vi "Measure vs B2Dv14.vi"() -> ()   [LabVIEW 2009]
doc: "This VI is an example operator panel.\n\nThe VI contains a table for the field values that may be configured manually, or loaded by checking the \"Prompt for File\" box. The data file should contain 3 columns of data, with each column delimited by a tab character.\n\nBefore the VI is executed, set the desired field units and coordinate system. Once the VI is started, follow the directions in the STATUS indicator to operate. Once a field value is achieved, it will be held indefinitely with no user intervention.\n\nThe present field is displayed in the selected units and coordinate system. The present field is queried once per second.\n\nIf a field point is specified that is outside the limits for the magnet, the VI will abort execution."
uses:
  <vilib>/Utility/file.llb/Read From Spreadsheet File (DBL).vi
panel:
  in  "Choose AH (2550 - 2700)":bool=TRUE
  in  "PID off":bool
  in  "Go to zero and SH off":bool=TRUE
  in  "Port Num- TRBridge":string="7"
  in  "GPIB SIM900":string="2"
  in  "TempSensor":bool
  in  "AH":bool=TRUE
  in  "GPIB HP 2":string="13"
  in  "Wait between \nVectors":bool
  in  "Change\nPID\n(DetermineSIMPID.vi)":bool
  in  "Wait between \nVectors (ms)":u32=3000
  in  "X Axis":enum16{"B", "phi"}(ring)
  in  "Y Axis":T1(ring)=enum."HP (V)2"
  out "measured data":dbl[][](array[numeric])
  out "XY Graph":T2(graph)
  in  "Notes:":string="test" caption="Notizen:"
  out "Messfile Refnum":refnum<file>
  in  "Measurement File":path=path "D:/UserData/fherzog/FH-4069-5B/test.txt"
  in  "Sample name:":string="FH-4069-5B"
  in  "HP 1":bool
  in  "GPIB HP":string="13"
  in  "HP 2":bool
  in  "LI 3":bool
  in  "GPIB L 3":string="8"
  in  "LI 2":bool
  in  "GPIB L 2":string="8"
  in  "LI 1":bool
  in  "GPIB L 1":string="8"
  out "Number of lines":i32=4
  in  "Operation":u16(ring)=1 items=["Stepwise", "Continous"]
  out "Ramp Rate along Vector (T/min)":dbl=0.060000000000000005 format="%.3f"
  out "Current Ramp Rate Z (T/min)":dbl=0.05908831630883079 format="%.3f"
  out "Current Ramp Rate Y (T/min)":dbl=0.010419734919255939 format="%.3f"
  in  "User defined Ramp Rate (T/min)":bool=TRUE
  in  "User defined Ramp Rate (T/min)":dbl=0.06 format="%.3f"
  in  "Z-Axis Communications Config":T3={"GPIB address"=22, "GPIB bus"=1, "connection ID"=refnum, "IP"="111.111.111.1", "Active Comm Interface"=0, "Serial Port"="", "Programmer Type"=0} {"Programmer Type" items=["Model 430", "Model 420"]; "Active Comm Interface" items=["TCP/IP (Model 430 Only)", "RS232", "IEEE488"]}
  in  "Max Ramp Rate - Y Axis (A/s)":dbl=0.055 format="%.3f"
  in  "Max Ramp Rate - Z Axis (A/s)":dbl=0.19 format="%.3f"
  in  "Magnitude Limit (kG)":dbl=45.1 format="%.3f"
  in  "Y-Axis Communications Config":T3={"GPIB address"=22, "GPIB bus"=1, "connection ID"=refnum, "IP"="111.111.111.2", "Active Comm Interface"=0, "Serial Port"="", "Programmer Type"=0} {"Programmer Type" items=["Model 430", "Model 420"]; "Active Comm Interface" items=["TCP/IP (Model 430 Only)", "RS232", "IEEE488"]}
  out "Cartesian Display (T)":T4={"Y-Axis Field (T)"=-0.08586, "Z-Axis Field (T)"=0.49363} {"Z-Axis Field (T)" format="%.3f"; "Y-Axis Field (T)" format="%.3f"}
  in  "Starting index":i32=4
  in  "Normal color":u32(colorbox)=11711154
  in  "Highlight color":u32(colorbox)=16711680
  in  "Prompt for File?":bool
  out "Continue Execution?":bool=TRUE
  out "error out":T5
  in  "error in":T5
  out "STATUS":string="Holding at current vector. Set Ramping Mode to NEXT VECTOR to continue."
  in  "Ramping Control":u16(ring)=2 items=["NEXT VECTOR", "RAMPING", "HOLDING", "PAUSE", "ZERO"]
  out "Cartesian Display (kG)":T6 {"Z-Axis Field (kG)" format="%.3f"; "Y-Axis Field (kG)" format="%.3f"}
  in  "Field Values":string[][](table)=[["3.5", "100"], ["8.1", "100"], ["3.5", "100"], ["8.1", "100"]]
  out "Switch Heaters":bool=TRUE
  out "Polar Display (T)":T7 {"Field Magnitude (T)" format="%.3f"; "q (degrees)" format="%.3f"}
  out "Polar Display (kG)":T8 {"Field Magnitude (kG)" format="%.3f"; "q (degrees)" format="%.3f"}
  in  "Coordinate System":u16(ring)=1 items=["Cartesian", "Polar"]
  in  "Magnetic Field Units":u16(ring)=1 items=["kG", "Tesla"]
  # "kontinuirliche Messung mit PID off bei 0, geht nur im Cartesian mode!"
  # "Measurement Display"
  # "Measurement Settings"
  # "Magnet Settings"
  # "Max Ramp Rate z: 1.27 T/min\nMax Ramp Rate y: 0.17 T/min"
  # "Devices"
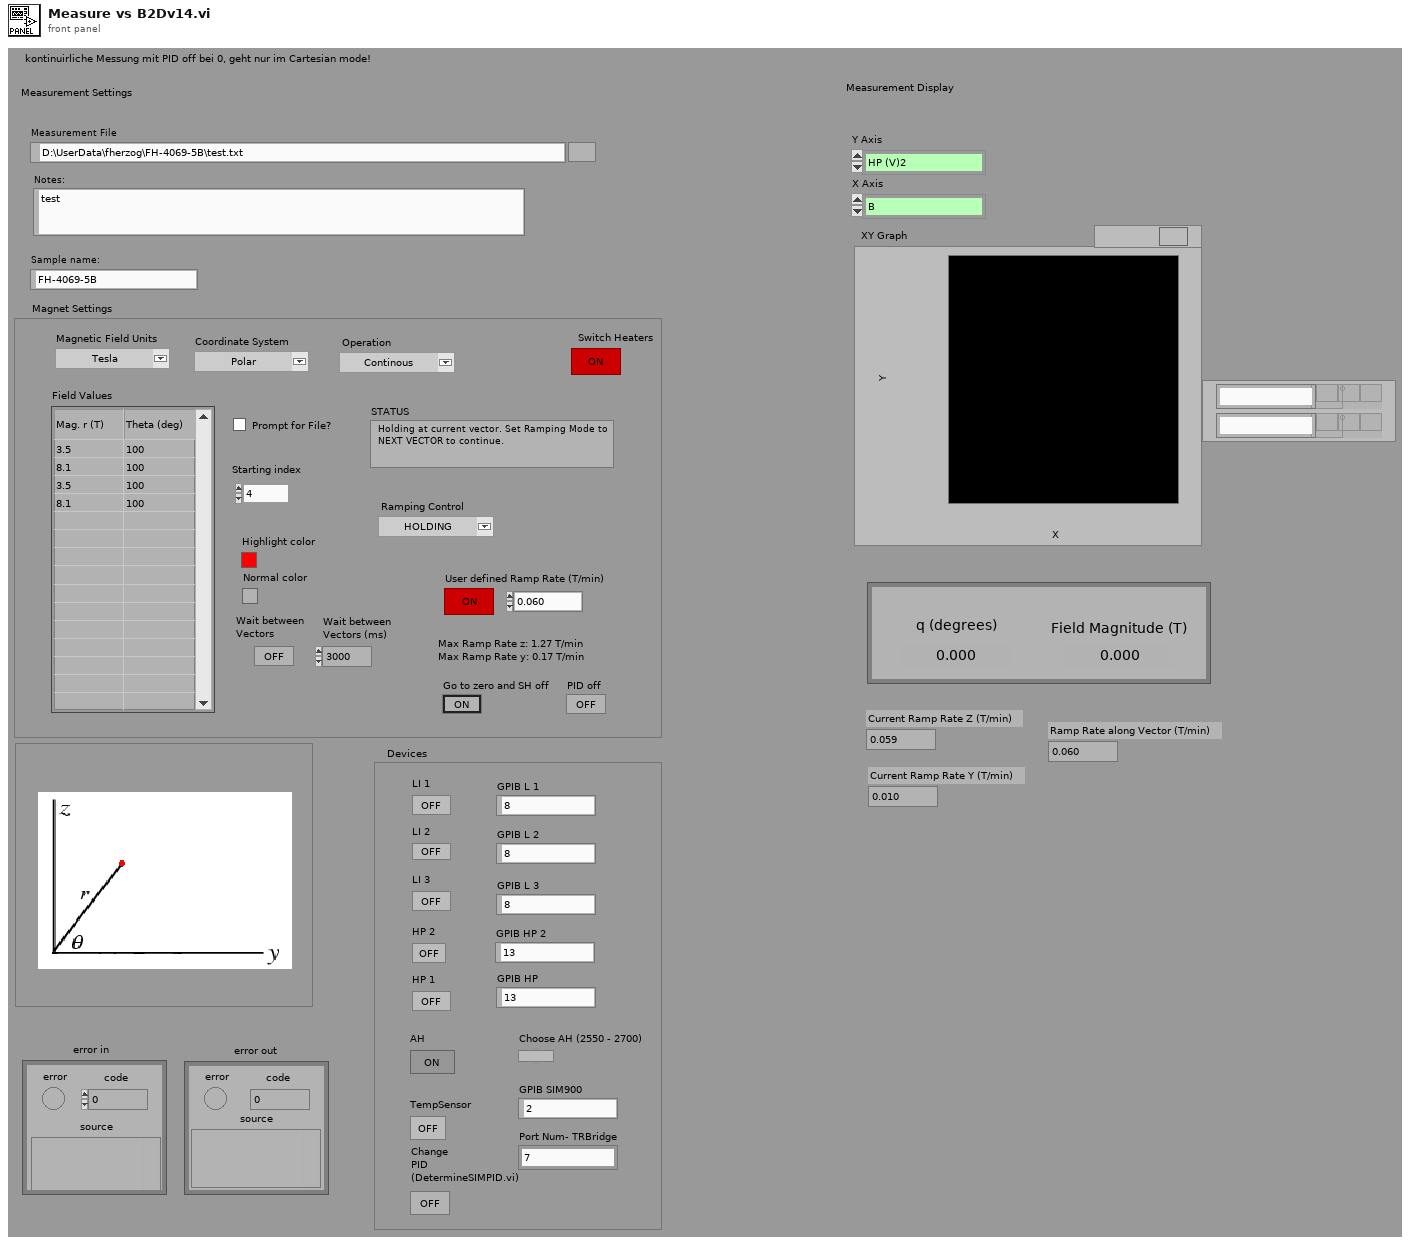
[diagram p1: front panel]
types:
  T1 = enum16{"B", "phi", "LI 1 Vx", "LI 1 Vy", "LI 2 Vx", "LI 2 Vy", "LI 3 Vx", "LI 3 Vy", "LI 4 Vx", "LI 4 Vy", "HP (V)", "HP (V)2", "AH C (pF)", "AH loss", "T (Ohms)", "Timestamp"}
  T2 = cluster{"measured data":dbl[], "measured data":dbl[]}
  T3 = cluster{"GPIB address":i16, "GPIB bus":i16, "connection ID":refnum<k5>, "IP":string, "Active Comm Interface":u16, "Serial Port":refnum<visa-resource-name>, "Programmer Type":u16}
  T4 = cluster{"Y-Axis Field (T)":dbl, "Z-Axis Field (T)":dbl}
  T5 = cluster{"error":bool, "code":i32, "source":string}
  T6 = cluster{"Y-Axis Field (kG)":dbl, "Z-Axis Field (kG)":dbl}
  T7 = cluster{"q (degrees)":dbl, "Field Magnitude (T)":dbl}
  T8 = cluster{"q (degrees)":dbl, "Field Magnitude (kG)":dbl}
  T9 = enum16{"", "RAMPING", "HOLDING", "PAUSED", "MANUAL UP", "MANUAL DOWN", "ZEROING CURRENT", "QUENCH DETECTED", "HEATING SWITCH"}
  T10 = enum16{"", "RAMPING", "HOLDING", "PAUSED", "MANUAL UP", "MANUAL DOWN", "ZEROING CURRENT", "QUENCH DETECTED", "HEATING SWITCH", "AT ZER0", "COOLING SWITCH"}
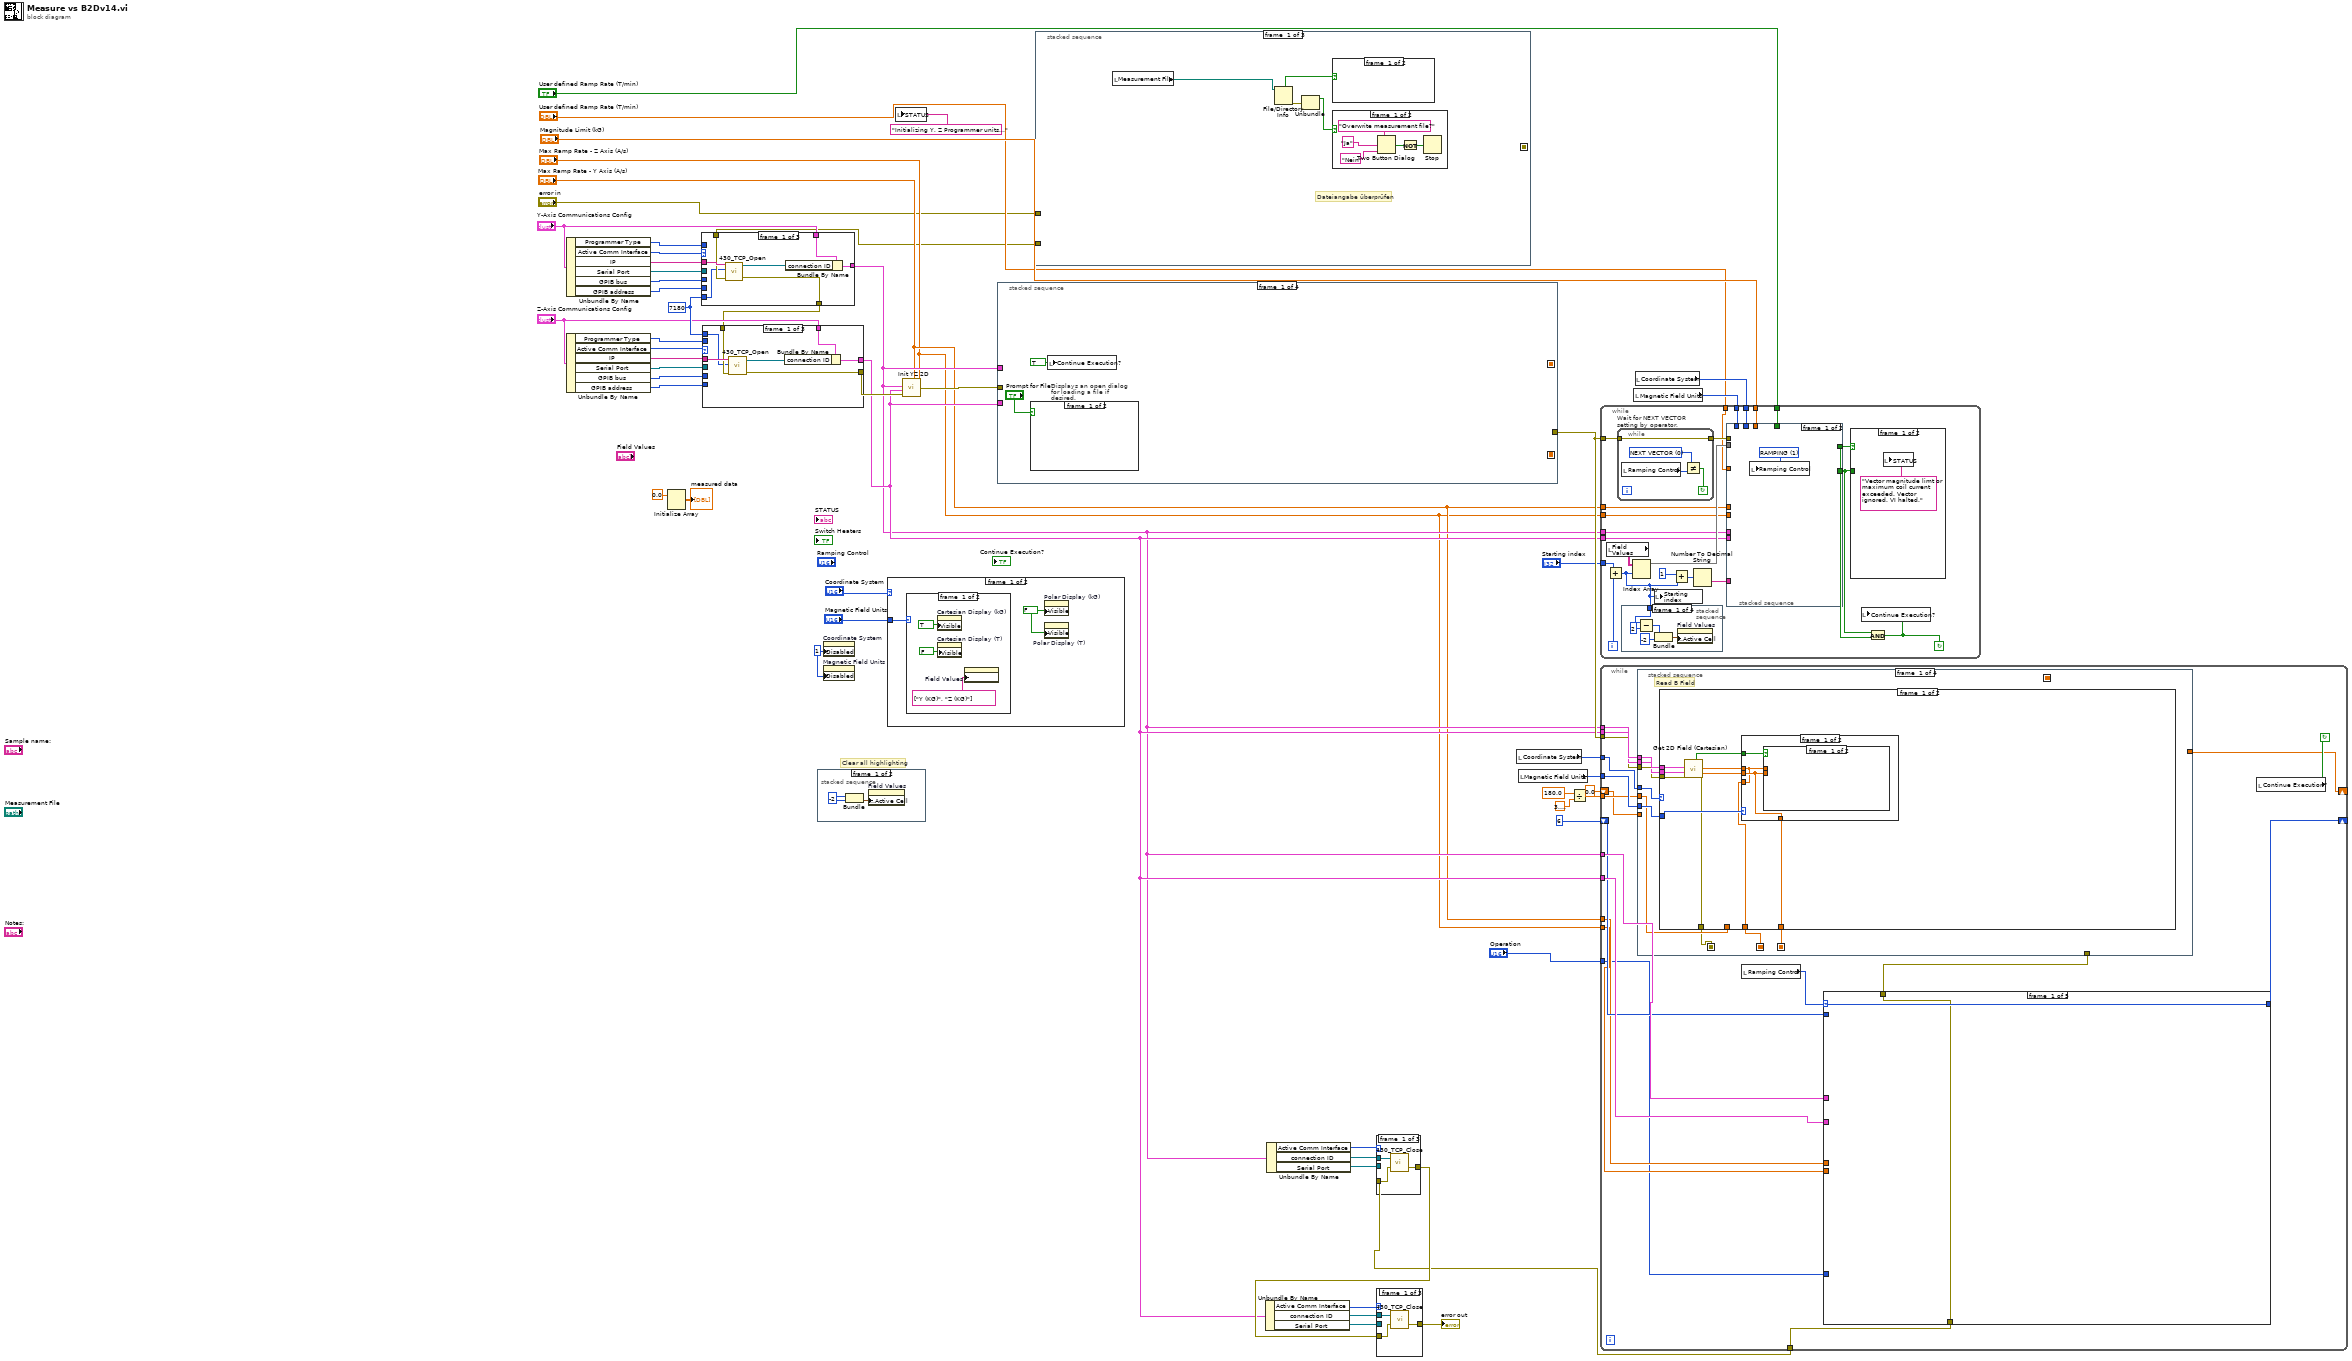
[diagram p0: block diagram]
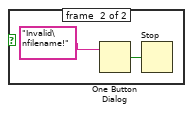
[diagram p3: hidden frame]
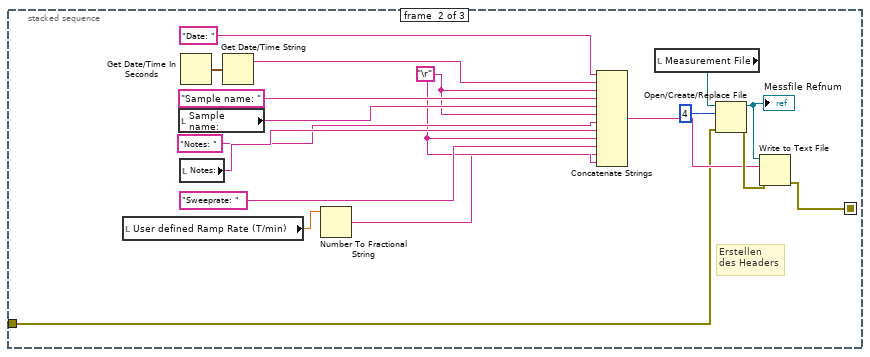
[diagram p4: hidden frame]
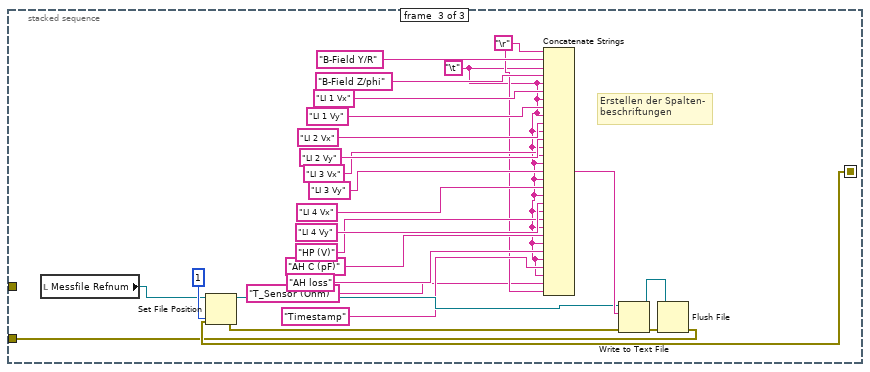
[diagram p5: hidden frame]
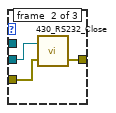
[diagram p6: hidden frame]
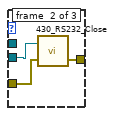
[diagram p8: hidden frame]
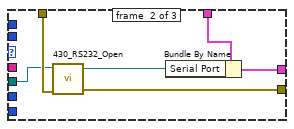
[diagram p10: hidden frame]
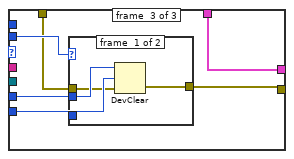
[diagram p11: hidden frame]
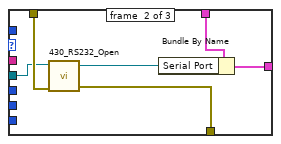
[diagram p13: hidden frame]
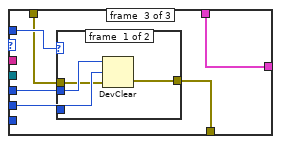
[diagram p14: hidden frame]
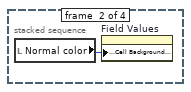
[diagram p16: hidden frame]
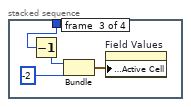
[diagram p17: hidden frame]
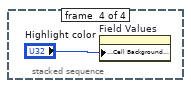
[diagram p18: hidden frame]
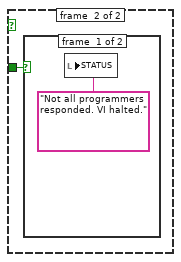
[diagram p19: hidden frame]
diagram:
  w39 = 7180 ("TCP Port")
  w52 = u8 1 ("Write Attribute")
  # "Clear all highlighting"
  n1 = Unbundle By Name("Z-Axis Communications Config") -> ("Programmer Type"=w15:u16, "Active Comm Interface"=w38:u16, "IP"=w35:string, "Serial Port"=w34:refnum<visa-resource-name>, "GPIB bus"=w14:i16, "GPIB address"=w13:i16)
  n2 = Unbundle By Name("Y-Axis Communications Config") -> ("Programmer Type"=w9:u16, "Active Comm Interface"=w37:u16, "IP"=w36:string, "Serial Port"=w33:refnum<visa-resource-name>, "GPIB bus"=w10:i16, "GPIB address"=w11:i16)
  n3 = Initialize Array(0.0 ("element")) -> (→"measured data":dbl[][])  [unwired: 2 in]
  n4 = stacked-sequence {
    frame #0 {
      w55 = -2
      n5 = Bundle(w55, w55) -> (w56:cluster{i32, i32})  [unwired: 1 in]
      n6 = property on="Field Values" class="Tbl (strict)"("Active Cell:Active Cell"=w56) -> ()  [unwired: 2 in, 2 out]
    }
    frame #1 {
      n7 = property on="Field Values" class="Tbl (strict)"("Active Cell:Cell Background Color"="Normal color") -> ()  [unwired: 2 in, 2 out]
    }
  }
  n8 = property on="Coordinate System" class="Ring (strict)"("Disabled"=w52) -> ()  [unwired: 2 in, 2 out]
  n9 = property on="Magnetic Field Units" class="Ring (strict)"("Disabled"=w52) -> ()  [unwired: 2 in, 2 out]
  n10 = case shown="1" "Coordinate System" {
    tunnel: "Magnetic Field Units" -> [w59 w67]
    frame #0 {
      w58 = FALSE ("Write Attribute")
      (unwired) FALSE ("Write Attribute")
      (unwired) TRUE ("Write Attribute")
      n11 = case shown="1" w59 {
        frame #0 {
          n12 = property on="Cartesian Display (kG)" class="Cluster (strict)"("Visible"=TRUE ("Write Attribute")) -> ()  [unwired: 2 in, 2 out]
          n13 = property on="Cartesian Display (T)" class="Cluster (strict)"("Visible"=FALSE ("Write Attribute")) -> ()  [unwired: 2 in, 2 out]
          n14 = property on="Field Values" class="Tbl (strict)"("Column Header Strings[]"=string[] ["Y (KG)", "Z (KG)"] ("Write Attribute")) -> ()  [unwired: 2 in, 2 out]
        }
        frame #1 {
          n15 = property on="Cartesian Display (kG)" class="Cluster (strict)"("Visible"=FALSE ("Write Attribute")) -> ()  [unwired: 2 in, 2 out]
          n16 = property on="Cartesian Display (T)" class="Cluster (strict)"("Visible"=TRUE ("Write Attribute")) -> ()  [unwired: 2 in, 2 out]
          n17 = property on="Field Values" class="Tbl (strict)"("Column Header Strings[]"=string[] ["Y (T)", "Z (T)"] ("Write Attribute")) -> ()  [unwired: 2 in, 2 out]
        }
      }
      n18 = property on="Polar Display (kG)" class="Clust (strict)"("Visible"=w58) -> ()  [unwired: 2 in, 2 out]
      n19 = property on="Polar Display (T)" class="Clust (strict)"("Visible"=w58) -> ()  [unwired: 2 in, 2 out]
    }
    frame #1 {
      (unwired) FALSE ("Write Attribute")
      (unwired) TRUE ("Write Attribute")
      w66 = FALSE ("Write Attribute")
      n20 = case shown="1" w67 {
        frame #0 {
          n21 = property on="Polar Display (kG)" class="Clust (strict)"("Visible"=TRUE ("Write Attribute")) -> ()  [unwired: 2 in, 2 out]
          n22 = property on="Polar Display (T)" class="Clust (strict)"("Visible"=FALSE ("Write Attribute")) -> ()  [unwired: 2 in, 2 out]
          n23 = property on="Field Values" class="Tbl (strict)"("Column Header Strings[]"=string[] ["Mag. r (KG)", "Theta (deg)"] ("Write Attribute")) -> ()  [unwired: 2 in, 2 out]
        }
        frame #1 {
          n24 = property on="Polar Display (kG)" class="Clust (strict)"("Visible"=FALSE ("Write Attribute")) -> ()  [unwired: 2 in, 2 out]
          n25 = property on="Polar Display (T)" class="Clust (strict)"("Visible"=TRUE ("Write Attribute")) -> ()  [unwired: 2 in, 2 out]
          n26 = property on="Field Values" class="Tbl (strict)"("Column Header Strings[]"=string[] ["Mag. r (T)", "Theta (deg)"] ("Write Attribute")) -> ()  [unwired: 2 in, 2 out]
        }
      }
      n27 = property on="Cartesian Display (kG)" class="Cluster (strict)"("Visible"=w66) -> ()  [unwired: 2 in, 2 out]
      n28 = property on="Cartesian Display (T)" class="Cluster (strict)"("Visible"=w66) -> ()  [unwired: 2 in, 2 out]
    }
  }
  n29 = local write "STATUS"("Initializing Y, Z Programmer units..." ("STATUS")) -> ()
  n30 = stacked-sequence {
    seq-local: [_ w85 _] -> [_ _ w110]
    tunnel: "error in" -> [_ w86 _]
    tunnel: [_ _ w109] -> w4
    frame #0 {
      # "Dateiangabe überprüfen"
      n31 = local read "Measurement File"() -> (w77:path)
      n32 = File/Directory Info(path=w77) -> (directory=w75:bool, error out=w76:errorcluster)  [unwired: 1 in, 5 out]
      n33 = Unbundle(w76) -> ("status"=w74:bool)  [unwired: 2 out]
      n34 = case shown="False" w75 {
        frame #0 {
        }
        frame #1 {
          n35 = One Button Dialog(message="Invalid\nfilename!") -> (true=w83:bool)  [unwired: 1 in]
          n36 = Stop(stop? (T)=w83) -> ()
        }
      }
      n37 = case shown="False" w74 {
        frame #0 {
          n38 = Two Button Dialog(message="Overwrite measurement file?", 1:"Nein", 2:"Ja") -> (T button?=w79:bool)
          n39 = Not(x=w79) -> (.not. x?=w78:bool)
          n40 = Stop(stop? (T)=w78) -> ()
        }
        frame #1 {
        }
      }
    }
    frame #1 {
      w89 = "\r"
      # "Erstellen\ndes Headers"
      n41 = local read "User defined Ramp Rate (T/min)"() -> (w88:dbl)
      n42 = local read "Sample name:"() -> (w95:string)
      n43 = local read "Notes:"() -> (w97:string)
      n44 = Get Date/Time In Seconds() -> (seconds since 1Jan1904=w91:timestamp)
      n45 = Get Date/Time String(seconds (now)=w91) -> (date string=w93:string)  [unwired: 2 in, 1 out]
      n46 = Number To Fractional String(number=w88) -> (F-format string=w87:string)  [unwired: 3 in]
      n47 = Concatenate Strings("Date: ", w93, w89, "Sample name: ", w95, w89, "Notes: ", w97, w89, "Sweeprate: ", w87, w89) -> (w101:string)
      n48 = local read "Measurement File"() -> (w98:path)
      n49 = Open/Create/Replace File(file path (use dialog)=w98, error in=w86, operation (0:open)=4) -> (refnum out=w100:refnum<file>, error out=w102:errorcluster)  [unwired: 3 in, 1 out]
      "Messfile Refnum" <- w100
      n50 = Write to Text File(file (use dialog)=w100, text=w101, error in=w102) -> (error out=w85:errorcluster)  [unwired: 1 in, 2 out]
    }
    frame #2 {
      w104 = "\t"
      w105 = "\r"
      # "Erstellen der Spalten-\nbeschriftungen"
      n51 = local read "Messfile Refnum"() -> (w117:refnum<file>)
      n52 = Set File Position(refnum=w117, from (0:start)=1, error in=w110) -> (refnum out=w123:refnum<file>, error out=w125:errorcluster)  [unwired: 1 in]
      n53 = Concatenate Strings(w105, "B-Field Y/R", w104, "B-Field Z/phi", w104, "LI 1 Vx", w104, "LI 1 Vy", w104, "LI 2 Vx", w104, "LI 2 Vy", w104, "LI 3 Vx", w104, "LI 3 Vy", w104, "LI 4 Vx", w104, "LI 4 Vy", w104, "HP (V)", w104, "AH C (pF)" ("string"), w104, "AH loss" ("string"), w104, "Timestamp", w104, "T_Sensor (Ohm)" ("string"), w105) -> (w124:string)
      n54 = Write to Text File(file (use dialog)=w123, text=w124, error in=w125) -> (refnum out=w127:refnum<file>, error out=w126:errorcluster)  [unwired: 1 in, 1 out]
      n55 = Flush File(refnum=w127, error in=w126) -> (error out=w109:errorcluster)  [unwired: 1 out]
    }
  }
  n56 = case shown="0, Default" w37 {
    tunnel: w36 -> [w135 _ _]
    tunnel: w4 -> [w134 w141 w143]
    tunnel: "Y-Axis Communications Config" -> [w133 w136 w147]
    tunnel: [w131 w139 w147] -> w22
    tunnel: [w130 w140 w142] -> w12
    tunnel: w39 -> [w129 _ _]
    tunnel: w33 -> [_ w137 _]
    tunnel: w11 -> [_ _ w146]
    tunnel: w10 -> [_ _ w145]
    tunnel: w9 -> [_ _ w144]
    frame #0 {
      n57 = call <userlib>:"430_TCP_Open.vi"("IP Address"=w135, "TCP Port"=w129, "error in (no error)"=w134) -> ("connection ID"=w132:refnum<k5>, "error out"=w130:errorcluster)  [unwired: 3 in, 1 out]
      n58 = Bundle By Name(cluster=w133, "connection ID"=w132) -> (w131:T3)
    }
    frame #1 {
      n59 = call <userlib>:"430_RS232_Open.vi"("VISA resource name"=w137, "error in (no error)"=w141) -> ("VISA resource name out"=w138:refnum<visa-resource-name>, "error out"=w140:errorcluster)  [unwired: 5 in]
      n60 = Bundle By Name(cluster=w136, "Serial Port"=w138) -> (w139:T3)
    }
    frame #2 {
      n61 = case shown="1" w144 {
        tunnel: w145 -> [w151 _]
        tunnel: w146 -> [w150 _]
        tunnel: w143 -> [w149 w152]
        tunnel: [w148 w152] -> w142
        frame #0 {
          n62 = DevClear(2:w149, 3:w150, 4:w151) -> (0:w148:errorcluster)  [unwired: 1 out]
        }
        frame #1 {
        }
      }
    }
  }
  n63 = case shown="0, Default" w38 {
    tunnel: w35 -> [w159 _ _]
    tunnel: w12 -> [w158 w165 w167]
    tunnel: [w157 w164 w166] -> w32
    tunnel: "Z-Axis Communications Config" -> [w156 w162 w171]
    tunnel: [w154 w163 w171] -> w23
    tunnel: w39 -> [w153 _ _]
    tunnel: w34 -> [_ w160 _]
    tunnel: w15 -> [_ _ w170]
    tunnel: w14 -> [_ _ w169]
    tunnel: w13 -> [_ _ w168]
    frame #0 {
      n64 = call <userlib>:"430_TCP_Open.vi"("IP Address"=w159, "TCP Port"=w153, "error in (no error)"=w158) -> ("connection ID"=w155:refnum<k5>, "error out"=w157:errorcluster)  [unwired: 3 in, 1 out]
      n65 = Bundle By Name(cluster=w156, "connection ID"=w155) -> (w154:T3)
    }
    frame #1 {
      n66 = call <userlib>:"430_RS232_Open.vi"("VISA resource name"=w160, "error in (no error)"=w165) -> ("VISA resource name out"=w161:refnum<visa-resource-name>, "error out"=w164:errorcluster)  [unwired: 5 in]
      n67 = Bundle By Name(cluster=w162, "Serial Port"=w161) -> (w163:T3)
    }
    frame #2 {
      n68 = case shown="0, Default" w170 {
        tunnel: w169 -> [w175 _]
        tunnel: w168 -> [w174 _]
        tunnel: w167 -> [w173 w176]
        tunnel: [w172 w176] -> w166
        frame #0 {
          n69 = DevClear(2:w173, 3:w174, 4:w175) -> (0:w172:errorcluster)  [unwired: 1 out]
        }
        frame #1 {
        }
      }
    }
  }
  n70 = call <userlib>:"Init YZ 2D.vi"("Max Ramp Rate Z-axis"="Max Ramp Rate - Z Axis (A/s)", "Max Ramp Rate Y-axis"="Max Ramp Rate - Y Axis (A/s)", "error in"=w32, "Z-Axis Communications Config"=w23, "Y-Axis Communications Config"=w22) -> ("error out"=w50:T5)  [unwired: 5 in]
  n71 = stacked-sequence {
    seq-local: [_ w184 _ _] -> [_ _ w231 _]
    seq-local: [_ w183 _ _] -> [_ _ w230 _]
    tunnel: w23 -> [_ w186 _ _]
    tunnel: w50 -> [_ w187 _ _]
    tunnel: [_ w182 _ _] -> w46
    tunnel: w22 -> [_ w185 _ _]
    frame #0 {
      n72 = case "Displays an open dialog for loading a file if desired." shown="True" "Prompt for File?" {
        frame #0 {
        }
        frame #1 {
          n73 = call-poly <vilib>:"Read From Spreadsheet File.vi"() -> ("all rows"=w181:dbl[][])  [unwired: 7 in, 4 out]
          n74 = Number To Fractional String(number=w181, precision (6)=i16 4) -> (F-format string=w180:string[][])  [unwired: 2 in]
          n75 = local write "Field Values"(w180) -> ()
        }
      }
      n76 = local write "Continue Execution?"(TRUE ("Continue Execution?")) -> ()
    }
    frame #1 {
      w195 = u16 3 items=["NEXT VECTOR", "RAMPING", "HOLDING", "PAUSE", "ZERO"] ("Ramping Control")
      n77 = call <userlib>:"Get Switch Present.vi"("error in"=w187, "Communications Config"=w185) -> ("error out"=w191:T5, "Switch Present?"=w192:bool)
      n78 = case shown="True" w192 {
        tunnel: w191 -> [w213 w222]
        tunnel: w185 -> [_ w215]
        tunnel: [0.0 w219] -> w183
        tunnel: [w213 w221] -> w190
        frame #0 {
        }
        frame #1 {
          n79 = call <userlib>:"Get Switch Heater Time.vi"("error in"=w222, "Communications Config"=w215) -> ("error out"=w218:T5, "Switch Heating Time (secs)"=w220:dbl)
          n80 = call <userlib>:"Get Switch Heater.vi"("error in"=w218, "Communications Config"=w215) -> ("error out"=w217:T5, "Switch Heater Indicator"=w216:bool)
          n81 = case shown="False" w216 {
            tunnel: [w227 w228] -> w221
            tunnel: w220 -> [w225 _]
            tunnel: [w225 0.0] -> w219
            tunnel: w217 -> [w223 w228]
            tunnel: w215 -> [w224 _]
            frame #0 {
              n82 = call <userlib>:"Set Switch Heater.vi"("error in"=w223, "Switch Heater Control"=TRUE, "Communications Config"=w224) -> ("error out"=w227:T5)
            }
            frame #1 {
            }
          }
        }
      }
      n83 = call <userlib>:"Get Switch Present.vi"("error in"=w190, "Communications Config"=w186) -> ("error out"=w188:T5, "Switch Present?"=w189:bool)
      n84 = case shown="True" w189 {
        tunnel: w188 -> [w196 w205]
        tunnel: w186 -> [_ w198]
        tunnel: [0.0 w202] -> w184
        tunnel: [w196 w204] -> w182
        frame #0 {
        }
        frame #1 {
          n85 = call <userlib>:"Get Switch Heater Time.vi"("error in"=w205, "Communications Config"=w198) -> ("error out"=w201:T5, "Switch Heating Time (secs)"=w203:dbl)
          n86 = call <userlib>:"Get Switch Heater.vi"("error in"=w201, "Communications Config"=w198) -> ("error out"=w200:T5, "Switch Heater Indicator"=w199:bool)
          n87 = case shown="False" w199 {
            tunnel: [w206 w211] -> w204
            tunnel: w203 -> [w209 _]
            tunnel: [w209 0.0] -> w202
            tunnel: w200 -> [w207 w211]
            tunnel: w198 -> [w208 _]
            frame #0 {
              n88 = call <userlib>:"Set Switch Heater.vi"("error in"=w207, "Switch Heater Control"=TRUE, "Communications Config"=w208) -> ("error out"=w206:T5)
            }
            frame #1 {
            }
          }
        }
      }
      n89 = local write "Ramping Control"(w195) -> ()
      n90 = local write "Switch Heaters"(TRUE ("Switch Heater Control")) -> ()
      n91 = property on="Switch Heaters" class="Boolean (strict)"("Disabled"=u8 1 ("Write Attribute")) -> ()  [unwired: 2 in, 2 out]
    }
    frame #2 {
      n92 = Max & Min(x=w231, y=w230) -> (max(x,y)=w232:dbl)  [unwired: 1 out]
      n93 = local write "STATUS"("Heating switches..." ("STATUS")) -> ()
      n94 = Add(x=w232, y=2) -> (x+y=w236:dbl)
      n95 = property on="Ramping Control" class="Ring (strict)"("Disabled"=u8 1 ("Write Attribute")) -> ()  [unwired: 2 in, 2 out]
      n96 = Multiply(x=w236, y=1000) -> (x*y=w235:dbl)
      n97 = Wait (ms)(milliseconds to wait=w235) -> ()  [unwired: 1 out]
    }
    frame #3 {
      n98 = property on="Ramping Control" class="Ring (strict)"("Disabled"=u8 0 ("Write Attribute")) -> ()  [unwired: 2 in, 2 out]
      n99 = local write "STATUS"("Ready to ramp to first vector. Set Ramping Mode to NEXT VECTOR to begin." ("STATUS")) -> ()
      n100 = local read "Field Values"() -> (w241:string[][])
      n101 = Array Size(array=w241) -> (size(s)=w240:i32[])
      n102 = Index Array(array=w240, index=0) -> (element=→"Number of lines":i32)
    }
  }
  n103 = Unbundle By Name(w23) -> ("Active Comm Interface"=w29:u16, "connection ID"=w28:refnum<k5>, "Serial Port"=w27:refnum<visa-resource-name>)
  n104 = Unbundle By Name(w22) -> ("Active Comm Interface"=w30:u16, "connection ID"=w26:refnum<k5>, "Serial Port"=w25:refnum<visa-resource-name>)
  n105 = local read "Coordinate System"() -> (w47:u16)
  n106 = local read "Magnetic Field Units"() -> (w45:u16)
  n107 = Divide(x=180.0, y=3.141592653589793) -> (x/y=w42:dbl)
  n108 = while {
    shift-left: u16 6 ("Ramping Control") -> [w251]
    shift-right: [w252] -> _
    tunnel: [w254] -> w24
    tunnel: w23 -> [w255]
    tunnel: w22 -> [w256]
    tunnel: w42 -> [w258]
    tunnel: w45 -> [w259]
    tunnel: w46 -> [w260]
    tunnel: w23 -> [w261]
    tunnel: w22 -> [w262]
    tunnel: w47 -> [w263]
    tunnel: "Max Ramp Rate - Y Axis (A/s)" -> [w250]
    tunnel: "Max Ramp Rate - Z Axis (A/s)" -> [w249]
    tunnel: "Operation" -> [w248]
    shift-right: [w246] -> _
    shift-left: 0.0 -> [w245]
    stop <- w253 continue-if-true
    n109 = stacked-sequence {
      seq-local: [w266 _ _ _] -> [_ _ w391 _]
      seq-local: [w265 _ _ _] -> [_ w339 w388 _]
      seq-local: [w264 _ _ _] -> [_ w340 w389 _]
      seq-local: [_ _ w376 _] -> [_ _ _ w473]
      tunnel: w263 -> [w272 _ _ w471]
      tunnel: w262 -> [w271 _ _ _]
      tunnel: w261 -> [w270 _ _ _]
      tunnel: w260 -> [w269 _ _ _]
      tunnel: w259 -> [w268 _ _ _]
      tunnel: w258 -> [w267 _ _ _]
      tunnel: [_ _ w390 _] -> w247
      tunnel: [_ w342 _ _] -> w246
      tunnel: w245 -> [_ w341 _ _]
      frame #0 {
        # "Read B Field"
        n110 = case shown="0, Default" w272 {
          tunnel: w271 -> [w282 w305]
          tunnel: w270 -> [w281 w304]
          tunnel: w269 -> [w280 w303]
          tunnel: w268 -> [w279 w302]
          tunnel: w267 -> [_ w301]
          tunnel: [w275 w300] -> w266
          tunnel: [w274 w298] -> w265
          tunnel: [w273 w299] -> w264
          frame #0 {
            n111 = call <userlib>:"Get 2D Field (Cartesian).vi"("Y-Axis Communications Config"=w282, "Z-Axis Communications Config"=w281, "error in"=w280) -> ("All Instruments Responded?"=w276:bool, "Y-Axis Field (kG)"=w278:dbl, "Z-Axis Field (kG)"=w277:dbl, "error out"=w275:T5)  [unwired: 2 in]
            n112 = case shown="0, Default" w279 {
              tunnel: w278 -> [w283 w291]
              tunnel: w277 -> [w284 w292]
              tunnel: w276 -> [w285 w294]
              tunnel: [w284 w290] -> w274
              tunnel: [w283 w289] -> w273
              frame #0 {
                n113 = case shown="True" w285 {
                  tunnel: w283 -> [_ w287]
                  tunnel: w284 -> [_ w286]
                  frame #0 {
                  }
                  frame #1 {
                    n114 = Bundle("Y-Axis Field (kG)"=w287, "Z-Axis Field (kG)"=w286) -> (→"Cartesian Display (kG)":T6)  [unwired: 1 in]
                  }
                }
              }
              frame #1 {
                w293 = 0.1 ("y")
                n115 = Multiply(x=w291, y=w293) -> (x*y=w289:dbl)
                n116 = Multiply(x=w292, y=w293) -> (x*y=w290:dbl)
                n117 = case shown="True" w294 {
                  tunnel: w289 -> [_ w297]
                  tunnel: w290 -> [_ w296]
                  frame #0 {
                  }
                  frame #1 {
                    n118 = Bundle(w297, w296) -> (→"Cartesian Display (T)":cluster{dbl, dbl})  [unwired: 1 in]
                  }
                }
              }
            }
          }
          frame #1 {
            n119 = stacked-sequence {
              tunnel: w305 -> [w316]
              tunnel: w304 -> [w315]
              tunnel: w303 -> [w314]
              tunnel: w302 -> [w313]
              tunnel: w301 -> [w310]
              tunnel: [w308] -> w300
              tunnel: [w307] -> w298
              tunnel: [w306] -> w299
              frame #0 {
                # "Field"
                n120 = call <userlib>:"Get 2D Field (Polar).vi"("Y-Axis Communications Config"=w316, "Z-Axis Communications Config"=w315, "error in"=w314) -> ("All Instruments Responded?"=w309:bool, "Radial (r) Field (kG)"=w312:dbl, "q (radians)"=w311:dbl, "error out"=w308:T5)  [unwired: 2 in]
                n121 = case shown="1" w313 {
                  tunnel: w312 -> [w318 w330]
                  tunnel: w311 -> [w320 w329]
                  tunnel: w310 -> [w319 w328]
                  tunnel: w309 -> [w321 w327]
                  tunnel: [w318 w325] -> w307
                  tunnel: [w317 w326] -> w306
                  frame #0 {
                    n122 = Multiply(x=w320, y=w319) -> (x*y=w317:dbl)
                    n123 = case shown="True" w321 {
                      tunnel: w318 -> [_ w322]
                      tunnel: w317 -> [_ w323]
                      frame #0 {
                      }
                      frame #1 {
                        n124 = Bundle(w323, "Radial (r) Field (kG)"=w322) -> (→"Polar Display (kG)":cluster{dbl, "Radial (r) Field (kG)":dbl})  [unwired: 1 in]
                      }
                    }
                  }
                  frame #1 {
                    n125 = Multiply(x=w330, y=0.1) -> (x*y=w326:dbl)
                    n126 = Multiply(x=w329, y=w328) -> (x*y=w325:dbl)
                    n127 = case shown="True" w327 {
                      tunnel: w326 -> [_ w332]
                      tunnel: w325 -> [_ w333]
                      frame #0 {
                      }
                      frame #1 {
                        n128 = Bundle(w333, w332) -> (→"Polar Display (T)":cluster{dbl, dbl})  [unwired: 1 in]
                      }
                    }
                  }
                }
              }
            }
          }
        }
      }
      frame #1 {
        # "Change PID"
        n129 = Square(x=w340) -> (x^2=w337:dbl)
        n130 = Square(x=w339) -> (x^2=w338:dbl)
        n131 = Add(x=w337, y=w338) -> (x+y=w336:dbl)
        n132 = Square Root(x=w336) -> (sqrt(x)=w335:dbl)
        n133 = case shown="False" "Change\nPID\n(DetermineSIMPID.vi)" {
          tunnel: w335 -> [_ w354]
          tunnel: [_ w350] -> w342
          tunnel: w341 -> [_ w352]
          frame #0 {
          }
          frame #1 {
            n134 = Absolute Value(x=w354) -> (abs(x)=w350:dbl)
            n135 = Less Or Equal?(x=w350, y=0.07 ("upper limit")) -> (x <= y?=w347:bool)
            n136 = Greater?(x=w352, y=0.07 ("upper limit")) -> (0:w348:bool)
            n137 = Not(x=w348) -> (.not. x?=w345:bool)
            n138 = Not(x=w347) -> (.not. x?=w346:bool)
            n139 = And(x=w348, y=w347) -> (x .and. y?=w353:bool)
            n140 = And(x=w345, y=w346) -> (x .and. y?=w344:bool)
            n141 = case shown="True" w353 {
              frame #0 {
              }
              frame #1 {
                n142 = stacked-sequence {
                  frame #0 {
                    n143 = call "SIM960Poff.vi"("off/on (0/1)"="0", "Port Num- PID"="1", "GPIB-Adress"="2") -> ()  [unwired: 9 in]
                  }
                  frame #1 {
                    n144 = call "SIM960Poff.vi"("off/on (0/1)"="0", "Port Num- PID"="3", "GPIB-Adress"="2") -> ()  [unwired: 9 in]
                  }
                  frame #2 {
                    n145 = call "SIM960ChangeSignP.vi"("Port Num- PID"="1", "GPIB-Adress"="2") -> ()  [unwired: 10 in]
                  }
                }
              }
            }
            n146 = case shown="True" w344 {
              frame #0 {
              }
              frame #1 {
                n147 = stacked-sequence {
                  frame #0 {
                    n148 = call "SIM960Poff.vi"("off/on (0/1)"="1", "Port Num- PID"="3", "GPIB-Adress"="2") -> ()  [unwired: 9 in]
                  }
                  frame #1 {
                    n149 = call "SIM960Poff.vi"("off/on (0/1)"="1", "Port Num- PID"="1", "GPIB-Adress"="2") -> ()  [unwired: 9 in]
                  }
                }
              }
            }
          }
        }
      }
      frame #2 {
        w375 = u16 2 items=["NEXT VECTOR", "RAMPING", "HOLDING", "PAUSE", "ZERO"] ("Ramping Control")
        # "Zeile in Datei schreiben"
        # "Read and Save Devices"
        n150 = stacked-sequence {
          tunnel: [w403 _ _ _ _ _ _ _] -> w387
          tunnel: [w402 _ _ _ _ _ _ _] -> w386
          tunnel: [_ w416 _ _ _ _ _ _] -> w383
          tunnel: [_ w414 _ _ _ _ _ _] -> w382
          tunnel: [_ _ w426 _ _ _ _ _] -> w381
          tunnel: [_ _ w425 _ _ _ _ _] -> w380
          tunnel: [_ _ _ w437 _ _ _ _] -> w379
          tunnel: [_ _ _ 0.0 _ _ _ _] -> w378
          tunnel: [_ _ _ _ w443 _ _ _] -> w377
          tunnel: [_ _ _ _ _ _ _ w467] -> w370
          tunnel: [_ _ _ _ _ w450 _ _] -> w372
          tunnel: [_ _ _ _ _ w449 _ _] -> w371
          tunnel: [_ _ _ _ _ _ w460 _] -> w369
          frame #0 {
            n151 = case shown="True" "LI 1" {
              tunnel: ["0" ("Antwort2") w410] -> w405
              tunnel: ["0" ("Antwort1") w409] -> w404
              frame #0 {
              }
              frame #1 {
                n152 = call "LI-Ansteuerung.vi"("Frage2"="OUTP? 2", "Frage1"="OUTP? 1", "address string"="GPIB L 1") -> ("Antwort2"=w410:string, "Antwort1"=w409:string)
              }
            }
            n153 = Fract/Exp String To Number(string=w405) -> (number=w402:dbl)  [unwired: 3 in, 1 out]
            n154 = Fract/Exp String To Number(string=w404) -> (number=w403:dbl)  [unwired: 3 in, 1 out]
          }
          frame #1 {
            n155 = case shown="True" "LI 2" {
              tunnel: [w419 w421] -> w415
              tunnel: [w419 w420] -> w417
              frame #0 {
                w419 = "0" ("Antwort1")
              }
              frame #1 {
                n156 = call "LI-Ansteuerung.vi"("Frage2"="OUTP? 2", "Frage1"="OUTP? 1", "address string"="GPIB L 2") -> ("Antwort2"=w421:string, "Antwort1"=w420:string)
              }
            }
            n157 = Fract/Exp String To Number(string=w415) -> (number=w414:dbl)  [unwired: 3 in, 1 out]
            n158 = Fract/Exp String To Number(string=w417) -> (number=w416:dbl)  [unwired: 3 in, 1 out]
          }
          frame #2 {
            n159 = case shown="True" "LI 3" {
              tunnel: [w430 w432] -> w427
              tunnel: [w430 w431] -> w428
              frame #0 {
                w430 = "0" ("Antwort1")
              }
              frame #1 {
                n160 = call "LI-Ansteuerung.vi"("Frage2"="OUTP? 2", "Frage1"="OUTP? 1", "address string"="GPIB L 3") -> ("Antwort2"=w432:string, "Antwort1"=w431:string)
              }
            }
            n161 = Fract/Exp String To Number(string=w428) -> (number=w426:dbl)  [unwired: 3 in, 1 out]
            n162 = Fract/Exp String To Number(string=w427) -> (number=w425:dbl)  [unwired: 3 in, 1 out]
          }
          frame #3 {
            n163 = case shown="True" "HP 2" {
              tunnel: [0.0 ("Voltage") w440] -> w437
              frame #0 {
              }
              frame #1 {
                n164 = call "HP-ReadVoltagev2.vi"("String"="meas:volt:dc? 10,0.001", "HP-Mulitmeter\nGPIB Address"="GPIB HP 2") -> ("Voltage"=w440:dbl)  [unwired: 9 in]
              }
            }
          }
          frame #4 {
            n165 = case shown="True" "HP 1" {
              tunnel: [0.0 ("Voltage") w447] -> w443
              frame #0 {
              }
              frame #1 {
                n166 = call "HP-ReadVoltagev2.vi"("String"="meas:volt:dc? 200,0.001", "HP-Mulitmeter\nGPIB Address"="GPIB HP") -> ("Voltage"=w447:dbl)  [unwired: 9 in]
              }
            }
          }
          frame #5 {
            n167 = case shown="True" "AH" {
              tunnel: [w452 w455] -> w449
              tunnel: [w452 w454] -> w450
              frame #0 {
                w452 = 0.0 ("Voltage")
              }
              frame #1 {
                n168 = case shown="False" "Choose AH (2550 - 2700)" {
                  tunnel: [w456 w459] -> w455
                  tunnel: [w457 w458] -> w454
                  frame #0 {
                    n169 = call "AHRead2700.vi"() -> ("loss"=w456:dbl, "capacitance"=w457:dbl)  [unwired: 9 in, 1 out]
                  }
                  frame #1 {
                    n170 = call "AHRead2550.vi"() -> ("loss"=w459:dbl, "capacitance"=w458:dbl)  [unwired: 9 in, 1 out]
                  }
                }
              }
            }
          }
          frame #6 {
            n171 = case shown="False" "TempSensor" {
              tunnel: [0.0 ("Voltage") w463] -> w460
              frame #0 {
              }
              frame #1 {
                n172 = call "Read_R_Bridge_new_v3.vi"("Port Num- TRBridge"="Port Num- TRBridge", "GPIB-Adress"="GPIB SIM900") -> ("R out"=w464:string)  [unwired: 8 in, 1 out]
                n173 = Fract/Exp String To Number(string=w464) -> (number=w463:dbl)  [unwired: 3 in, 1 out]
              }
            }
          }
          frame #7 {
            n174 = Get Date/Time In Seconds() -> (seconds since 1Jan1904=w468:timestamp)
            n175 = To Double Precision Float(number=w468) -> (double precision float=w467:dbl)
          }
        }
        n176 = local read "Ramping Control"() -> (w374:u16)
        n177 = Build Array(w389, w388, w387, w386, w383, w382, w380, w381, w379, w378, w377, w372, w371, w369, w370) -> (w376:dbl[])
        n178 = Array To Spreadsheet String(array=w376, 3:"%.8f" ("format string")) -> (spreadsheet string=w385:string)  [unwired: 1 in]
        n179 = Equal?(x=w374, y=w375) -> (x = y?=w373:bool)
        n180 = case shown="False" w373 {
          tunnel: w391 -> [w400 w401]
          tunnel: [w399 w401] -> w390
          tunnel: w385 -> [w398 _]
          frame #0 {
            n181 = local read "Messfile Refnum"() -> (w392:refnum<file>)
            n182 = Set File Position(refnum=w392, from (0:start)=1, error in=w400) -> (refnum out=w394:refnum<file>, error out=w395:errorcluster)  [unwired: 1 in]
            n183 = Write to Text File(file (use dialog)=w394, text=w398, error in=w395) -> (refnum out=w397:refnum<file>, error out=w396:errorcluster)  [unwired: 1 in, 1 out]
            n184 = Flush File(refnum=w397, error in=w396) -> (error out=w399:errorcluster)  [unwired: 1 out]
          }
          frame #1 {
          }
        }
      }
      frame #3 {
        n185 = local read "measured data"() -> (w474:dbl[][])
        n186 = Insert Into Array(array=w474, new element=w473) -> (w472:dbl[][])  [unwired: 2 in]
        n187 = case shown="0, Default" w471 {
          tunnel: w472 -> [w490 w504]
          tunnel: "Y Axis" -> [w492 w503]
          tunnel: "X Axis" -> [w480 w502]
          frame #0 {
            n188 = Index Array(array=w490, index (col)=1 ("disabled index (col)")) -> (element=w485:dbl[])  [unwired: 1 in]
            n189 = Index Array(array=w490, index (col)=0 ("disabled index (col)")) -> (element=w484:dbl[])  [unwired: 1 in]
            n190 = Square(x=w485) -> (x^2=w487:dbl[])
            n191 = Square(x=w484) -> (x^2=w488:dbl[])
            n192 = Index Array(array=w490, index (col)=w492) -> (element=w479:dbl[])  [unwired: 1 in]
            n193 = Divide(x=w485, y=w484) -> (x/y=w476:dbl[])
            n194 = Add(x=w488, y=w487) -> (x+y=w486:dbl[])
            n195 = Inverse Tangent(1:w476) -> (0:w475:dbl[])
            n196 = Square Root(x=w486) -> (sqrt(x)=w477:dbl[])
            n197 = Divide(x=w475, y=3.141592653589793) -> (x/y=w482:dbl[])
            n198 = Multiply(x=w482, y=180) -> (x*y=w478:dbl[])
            n199 = case shown="\"B\", Default" w480 {
              tunnel: w479 -> [w495 w498]
              tunnel: w478 -> [_ w497]
              tunnel: w477 -> [w494 _]
              frame #0 {
                n200 = Bundle(w494, "measured data"=w495) -> (w493:cluster{dbl[], "measured data":dbl[]})  [unwired: 1 in]
                n201 = local write "XY Graph"(w493) -> ()
              }
              frame #1 {
                n202 = Bundle(w497, "measured data"=w498) -> (w496:cluster{dbl[], "measured data":dbl[]})  [unwired: 1 in]
                n203 = local write "XY Graph"(w496) -> ()
              }
            }
          }
          frame #1 {
            n204 = Index Array(array=w504, index (col)=w502) -> (element=w501:dbl[])  [unwired: 1 in]
            n205 = Index Array(array=w504, index (col)=w503) -> (element=w500:dbl[])  [unwired: 1 in]
            n206 = Bundle("measured data"=w501, "measured data"=w500) -> (w499:T2)  [unwired: 1 in]
            n207 = local write "XY Graph"(w499) -> ()
          }
        }
        n208 = local write "measured data"(w472) -> ()
      }
    }
    n209 = local read "Ramping Control"() -> (w257:u16)
    n210 = case shown="1" w257 {
      selector: w257 -> [w506 w526 w611 w615 w630]
      tunnel: w256 -> [_ w511 _ w618 w635]
      tunnel: w255 -> [_ w510 _ w617 w634]
      tunnel: [w505 w508 w610 w616 w633] -> w254
      tunnel: [w506 w526 w611 w615 w630] -> w252
      tunnel: w251 -> [_ _ _ w614 w632]
      tunnel: w250 -> [_ _ _ _ w629]
      tunnel: w249 -> [_ _ _ _ w628]
      tunnel: w248 -> [_ w518 _ _ _]
      tunnel: w247 -> [w505 w514 w610 w612 w627]
      frame #0 {
      }
      frame #1 {
        w521 = T9."HOLDING" ("y")
        n211 = local read "Number of lines"() -> (w515:i32)
        n212 = local read "Starting index"() -> (w517:i32)
        n213 = call <userlib>:"Get Ramping Mode.vi"("Communications Config"=w511, "error in"=w514) -> ("Ramping Mode"=w524:T10, "error out"=w525:T5)  [unwired: 1 out]
        n214 = call <userlib>:"Get Ramping Mode.vi"("Communications Config"=w510, "error in"=w525) -> ("Ramping Mode"=w523:T10, "error out"=w509:T5)  [unwired: 1 out]
        n215 = Less?(x=w517, y=w515) -> (x < y?=w516:bool)
        n216 = Equal?(x=w524, y=w521) -> (x = y?=w520:bool)
        n217 = Equal?(x=w523, y=w521) -> (x = y?=w519:bool)
        n218 = Compound Arithmetic op=AND(w520, w519) -> (w522:bool)
        n219 = case shown="True" w522 {
          tunnel: w518 -> [_ w536]
          tunnel: w516 -> [_ w535]
          tunnel: "Wait between \nVectors (ms)" -> [_ w534]
          tunnel: "Wait between \nVectors" -> [_ w533]
          tunnel: w511 -> [_ w531]
          tunnel: w510 -> [_ w530]
          tunnel: w509 -> [w527 w529]
          tunnel: [w527 w528] -> w508
          tunnel: "Go to zero and SH off" -> [_ w532]
          frame #0 {
          }
          frame #1 {
            n220 = case shown="1" w536 {
              tunnel: w535 -> [_ w547]
              tunnel: w534 -> [_ w546]
              tunnel: w533 -> [_ w545]
              tunnel: w532 -> [_ w544]
              tunnel: w531 -> [_ w543]
              tunnel: w530 -> [_ w542]
              tunnel: w529 -> [w537 w541]
              tunnel: [w537 w540] -> w528
              frame #0 {
                w539 = u16 2 items=["NEXT VECTOR", "RAMPING", "HOLDING", "PAUSE", "ZERO"] ("Ramping Control")
                n221 = local write "STATUS"("Holding at current vector. Set Ramping Mode to NEXT VECTOR to continue." ("STATUS")) -> ()
                n222 = local write "Ramping Control"(w539) -> ()
              }
              frame #1 {
                # "Go to NEXT VECTOR automatically"
                n223 = case shown="False" w547 {
                  tunnel: w546 -> [_ w604]
                  tunnel: w545 -> [_ w603]
                  tunnel: w544 -> [w552 _]
                  tunnel: w543 -> [w551 _]
                  tunnel: w542 -> [w550 _]
                  tunnel: w541 -> [w549 w602]
                  tunnel: [w548 w602] -> w540
                  frame #0 {
                    n224 = case shown="True" w552 {
                      tunnel: [w553 w557] -> w548
                      tunnel: w551 -> [_ w556]
                      tunnel: w550 -> [_ w555]
                      tunnel: w549 -> [w553 w554]
                      frame #0 {
                      }
                      frame #1 {
                        n225 = stacked-sequence {
                          seq-local: [_ _ w574 _ _ _ _] -> [_ _ _ _ w595 _ _]
                          tunnel: [_ _ _ _ w593 _ _] -> w557
                          tunnel: w556 -> [_ w561 w573 _ _ _ _]
                          tunnel: w555 -> [_ w560 w572 _ _ _ _]
                          tunnel: w554 -> [_ _ w571 _ _ _ _]
                          frame #0 {
                            w558 = u16 2 items=["NEXT VECTOR", "RAMPING", "HOLDING", "PAUSE", "ZERO"] ("Ramping Control")
                            n226 = local write "STATUS"("Holding at current vector. Set Ramping Mode to NEXT VECTOR to continue." ("STATUS")) -> ()
                            n227 = local write "Ramping Control"(w558) -> ()
                          }
                          frame #1 {
                            w566 = u16 0 items=["kG", "Tesla"] ("Magnetic Field Units")
                            w565 = u16 0 items=["Cartesian", "Polar"] ("Coordinate System")
                            n228 = Build Array("0", "0") -> (w564:string[])
                            n229 = call <userlib>:"Set 2D Next Vector_entwurf.vi"("Coordinate System"=w565, "Magnetic Field Units"=w566, "Magnitude Limit (kG)"=45.0, "Y-Axis Communications Config"=w561, "Input Vector"=w564, "Z-Axis Communications Config"=w560, "User defined Ramp Rate (T/min)"=FALSE, "Max Ramp Rate - Y Axis (A/s)"=0.05, "Max Ramp Rate - Z Axis (A/s)"=0.15) -> ()  [unwired: 5 in, 6 out]
                          }
                          frame #2 {
                            n230 = while {
                              tunnel: [w578] -> w574
                              tunnel: w573 -> [w577]
                              tunnel: w572 -> [w576]
                              tunnel: w571 -> [w575]
                              stop <- w580 stop-if-true
                              w583 = T9."HOLDING" ("y")
                              n231 = call <userlib>:"Get Ramping Mode.vi"("Communications Config"=w577, "error in"=w575) -> ("Ramping Mode"=w584:T10, "error out"=w586:T5)  [unwired: 1 out]
                              n232 = call <userlib>:"Get Ramping Mode.vi"("Communications Config"=w576, "error in"=w586) -> ("Ramping Mode"=w585:T10, "error out"=w578:T5)  [unwired: 1 out]
                              n233 = Equal?(x=w584, y=w583) -> (x = y?=w582:bool)
                              n234 = Equal?(x=w585, y=w583) -> (x = y?=w581:bool)
                              n235 = Compound Arithmetic op=AND(w582, w581) -> (w580:bool)
                              n236 = Wait (ms)(milliseconds to wait=u32 1000) -> ()  [unwired: 1 out]
                            }
                          }
                          frame #3 {
                            n237 = case shown="True" "PID off" {
                              frame #0 {
                              }
                              frame #1 {
                                w590 = "0" ("off/on (0/1)")
                                w591 = "2" ("GPIB-Adress")
                                n238 = call "SIM960Poff.vi"("off/on (0/1)"=w590, "Port Num- PID"="3", "GPIB-Adress"=w591) -> ()  [unwired: 9 in]
                                n239 = call "SIM960Poff.vi"("off/on (0/1)"=w590, "Port Num- PID"="1", "GPIB-Adress"=w591) -> ()  [unwired: 9 in]
                              }
                            }
                            n240 = Wait (ms)(milliseconds to wait=u32 10000) -> ()  [unwired: 1 out]
                          }
                          frame #4 {
                            w596 = u16 1 items=["RAMP", "PAUSE", "MANUAL UP", "MANUAL DOWN", "ZERO"] ("Ramping Mode")
                            w597 = u16 1 items=["RAMP", "PAUSE", "MANUAL UP", "MANUAL DOWN", "ZERO"] ("Ramping Mode")
                            n241 = call <userlib>:"Set Ramping Mode.vi"("error in"=w595, "Ramping Mode"=w597) -> ("error out"=w594:T5)  [unwired: 1 in]
                            n242 = call <userlib>:"Set Ramping Mode.vi"("error in"=w594, "Ramping Mode"=w596) -> ("error out"=w593:T5)  [unwired: 1 in]
                          }
                          frame #5 {
                            n243 = call <userlib>:"430_TCP_PSoff.vi"("IP Address"="111.111.111.2", "Switch Heater Control"=FALSE) -> ()  [unwired: 5 in, 2 out]
                            n244 = call <userlib>:"430_TCP_PSoff.vi"("IP Address"="111.111.111.1", "Switch Heater Control"=FALSE) -> ()  [unwired: 5 in, 2 out]
                          }
                          frame #6 {
                          }
                        }
                      }
                    }
                  }
                  frame #1 {
                    n245 = stacked-sequence {
                      tunnel: w604 -> [w606 _]
                      tunnel: w603 -> [w605 _]
                      frame #0 {
                        n246 = case shown="True" w605 {
                          tunnel: w606 -> [_ w607]
                          frame #0 {
                          }
                          frame #1 {
                            n247 = Wait (ms)(milliseconds to wait=w607) -> ()  [unwired: 1 out]
                          }
                        }
                      }
                      frame #1 {
                        w609 = u16 0 items=["NEXT VECTOR", "RAMPING", "HOLDING", "PAUSE", "ZERO"] ("Ramping Control")
                        n248 = local write "Ramping Control"(w609) -> ()
                        n249 = local write "STATUS"("Go to NEXT VECTOR" ("STATUS")) -> ()
                      }
                    }
                  }
                }
              }
            }
          }
        }
      }
      frame #2 {
      }
      frame #3 {
        n250 = Not Equal?(x=w615, y=w614) -> (x != y?=w613:bool)
        n251 = case shown="False" w613 {
          tunnel: w618 -> [_ w626]
          tunnel: w617 -> [_ w625]
          tunnel: [w619 w623] -> w616
          tunnel: w612 -> [w619 w620]
          frame #0 {
          }
          frame #1 {
            w621 = u16 1 items=["RAMP", "PAUSE", "MANUAL UP", "MANUAL DOWN", "ZERO"] ("Ramping Mode")
            n252 = call <userlib>:"Set Ramping Mode.vi"("error in"=w620, "Ramping Mode"=w621, "Communications Config"=w626) -> ("error out"=w624:T5)
            n253 = call <userlib>:"Set Ramping Mode.vi"("error in"=w624, "Ramping Mode"=w621, "Communications Config"=w625) -> ("error out"=w623:T5)
            n254 = local write "STATUS"("All Programmers are PAUSED. Set Ramping Mode to NEXT VECTOR to continue." ("STATUS")) -> ()
          }
        }
      }
      frame #4 {
        n255 = Not Equal?(x=w630, y=w632) -> (x != y?=w631:bool)
        n256 = case shown="False" w631 {
          tunnel: w635 -> [_ w644]
          tunnel: w634 -> [_ w643]
          tunnel: [w636 w639] -> w633
          tunnel: w629 -> [_ w642]
          tunnel: w628 -> [_ w641]
          tunnel: w627 -> [w636 w637]
          frame #0 {
          }
          frame #1 {
            w638 = u16 4 items=["RAMP", "PAUSE", "MANUAL UP", "MANUAL DOWN", "ZERO"] ("Ramping Mode")
            n257 = local write "STATUS"("Zeroing vector." ("STATUS")) -> ()
            n258 = call <userlib>:"Set Ramping Mode.vi"("error in"=w637, "Ramping Mode"=w638, "Communications Config"=w644) -> ("error out"=w647:T5)
            n259 = call <userlib>:"Set Ramping Mode.vi"("error in"=w647, "Ramping Mode"=w638, "Communications Config"=w643) -> ("error out"=w640:T5)
            n260 = call <userlib>:"Set Current Ramp Rate.vi"("Communications Config"=w644, "Ramp Rate (A/sec)"=w642, "error in"=w640) -> ("error out"=w645:T5)  [unwired: 2 in]
            n261 = call <userlib>:"Set Current Ramp Rate.vi"("Communications Config"=w643, "Ramp Rate (A/sec)"=w641, "error in"=w645) -> ("error out"=w639:T5)  [unwired: 2 in]
          }
        }
      }
    }
    n262 = local read "Continue Execution?"() -> (w253:bool)
  }
  n263 = case shown="0, Default" w30 {
    tunnel: w26 -> [w650 _ _]
    tunnel: w24 -> [w649 w653 w654]
    tunnel: [w648 w652 w654] -> w31
    tunnel: w25 -> [_ w651 _]
    frame #0 {
      n264 = call <userlib>:"430_TCP_Close.vi"("error in (no error)"=w649, "connection ID"=w650) -> ("error out"=w648:errorcluster)  [unwired: 1 out]
    }
    frame #1 {
      n265 = call <userlib>:"430_RS232_Close.vi"("error in (no error)"=w653, "VISA resource name"=w651) -> ("error out"=w652:errorcluster)  [unwired: 1 in]
    }
    frame #2 {
    }
  }
  n266 = case shown="0, Default" w29 {
    tunnel: w28 -> [w657 _ _]
    tunnel: w31 -> [w656 w660 w661]
    tunnel: [w655 w659 w661] -> w21
    tunnel: w27 -> [_ w658 _]
    frame #0 {
      n267 = call <userlib>:"430_TCP_Close.vi"("error in (no error)"=w656, "connection ID"=w657) -> ("error out"=w655:errorcluster)  [unwired: 1 out]
    }
    frame #1 {
      n268 = call <userlib>:"430_RS232_Close.vi"("error in (no error)"=w660, "VISA resource name"=w658) -> ("error out"=w659:errorcluster)  [unwired: 1 in]
    }
    frame #2 {
    }
  }
  "error out" <- w21
  n269 = local read "Magnetic Field Units"() -> (w48:u16)
  n270 = local read "Coordinate System"() -> (w49:u16)
  n271 = while {
    tunnel: "Starting index" -> [w669]
    tunnel: w23 -> [w675]
    tunnel: w22 -> [w676]
    tunnel: w48 -> [w677]
    tunnel: w49 -> [w678]
    tunnel: w46 -> [w681]
    tunnel: "Max Ramp Rate - Y Axis (A/s)" -> [w665]
    tunnel: "Max Ramp Rate - Z Axis (A/s)" -> [w664]
    tunnel: "Magnitude Limit (kG)" -> [w666]
    tunnel: "User defined Ramp Rate (T/min)" -> [w663]
    tunnel: "User defined Ramp Rate (T/min)" -> [w662]
    i -> [w668]
    stop <- w670 continue-if-true
    n272 = local read "Field Values"() -> (w672:string[][])
    n273 = Add(x=w669, y=w668) -> (x+y=w667:i32)
    n274 = while "Wait for NEXT VECTOR setting by operator." {
      tunnel: [w685] -> w680
      tunnel: w681 -> [w685]
      stop <- w686 continue-if-true
      w684 = u16 0 items=["NEXT VECTOR", "RAMPING", "HOLDING", "PAUSE", "ZERO"] ("Ramping Control")
      n275 = local read "Ramping Control"() -> (w687:u16)
      n276 = Not Equal?(x=w684, y=w687) -> (x != y?=w686:bool)
    }
    n277 = stacked-sequence {
      tunnel: w667 -> [w689 _ w695 _]
      frame #0 {
        (unwired) -2
        n278 = Subtract(x=w689, y=2) -> (x-y=w692:i32)
        n279 = Bundle(w692, -2) -> (w690:cluster{i32, i32})  [unwired: 1 in]
        n280 = property on="Field Values" class="Tbl (strict)"("Active Cell:Active Cell"=w690) -> ()  [unwired: 2 in, 2 out]
      }
      frame #1 {
        n281 = local read "Normal color"() -> (w693:u32)
        n282 = property on="Field Values" class="Tbl (strict)"("Active Cell:Cell Background Color"=w693) -> ()  [unwired: 2 in, 2 out]
      }
      frame #2 {
        n283 = Decrement(x=w695) -> (x-1=w694:i32)
        n284 = Bundle(w694, -2) -> (w697:cluster{i32, i32})  [unwired: 1 in]
        n285 = property on="Field Values" class="Tbl (strict)"("Active Cell:Active Cell"=w697) -> ()  [unwired: 2 in, 2 out]
      }
      frame #3 {
        n286 = property on="Field Values" class="Tbl (strict)"("Active Cell:Cell Background Color"="Highlight color") -> ()  [unwired: 2 in, 2 out]
      }
    }
    n287 = Index Array(array=w672, index (row)=w667) -> (element=w679:string[])  [unwired: 1 in]
    n288 = local write "Starting index"(w667) -> ()
    n289 = Add(x=1, y=w667) -> (x+y=w682:i32)
    n290 = Number To Decimal String(number=w682) -> (decimal integer string=w671:string)  [unwired: 1 in]
    n291 = stacked-sequence {
      tunnel: [_ w723] -> w673
      tunnel: [_ w722] -> w674
      tunnel: w680 -> [_ w718]
      tunnel: w679 -> [_ w717]
      tunnel: w678 -> [_ w716]
      tunnel: w677 -> [_ w715]
      tunnel: w676 -> [_ w714]
      tunnel: w675 -> [_ w713]
      tunnel: w671 -> [_ w712]
      tunnel: w666 -> [_ w710]
      tunnel: w665 -> [_ w709]
      tunnel: w664 -> [_ w704]
      tunnel: w663 -> [_ w708]
      tunnel: w662 -> [_ w707]
      frame #0 {
        w702 = u16 1 items=["NEXT VECTOR", "RAMPING", "HOLDING", "PAUSE", "ZERO"] ("Ramping Control")
        n292 = local write "Ramping Control"(w702) -> ()
      }
      frame #1 {
        n293 = call <userlib>:"Set 2D Next Vector_entwurf.vi"("Coordinate System"=w716, "Magnetic Field Units"=w715, 3:"User defined Ramp Rate (T/min)"=w707, "Magnitude Limit (kG)"=w710, "Y-Axis Communications Config"=w714, "Input Vector"=w717, "Z-Axis Communications Config"=w713, 10:"User defined Ramp Rate (T/min)"=w708, "Max Ramp Rate - Y Axis (A/s)"=w709, "error in"=w718, "Max Ramp Rate - Z Axis (A/s)"=w704) -> ("Y-Axis Ramp Rate (T/min)"=→"Current Ramp Rate Y (T/min)":dbl, "Within Limits?"=w723:bool, "Ramp Rate along Vector (T/min)"=→"Ramp Rate along Vector (T/min)":dbl, "Z-Axis Ramp Rate (T/min)"=→"Current Ramp Rate Z (T/min)":dbl, "All Instruments Responded?"=w722:bool, "error out"=w711:T5)  [unwired: 3 in]
        n294 = Concatenate Strings("Ramping to field vector " ("STATUS"), w712, "..." ("STATUS")) -> (w719:string)
        n295 = local write "error in"(w711) -> ()
        n296 = local write "STATUS"(w719) -> ()
      }
    }
    n297 = case shown="True" w673 {
      tunnel: w674 -> [_ w700]
      frame #0 {
        n298 = local write "STATUS"("Vector magnitude limt or maximum coil current exceeded. Vector ignored. VI halted." ("STATUS")) -> ()
      }
      frame #1 {
        n299 = case shown="True" w700 {
          frame #0 {
            n300 = local write "STATUS"("Not all programmers responded. VI halted." ("STATUS")) -> ()
          }
          frame #1 {
          }
        }
      }
    }
    n301 = Compound Arithmetic op=AND(w674, w673) -> (w670:bool)
    n302 = local write "Continue Execution?"(w670) -> ()
  }
